vi "Write DAQmx Task Name.vi"(8 "error in (no error)":errorcluster, 10 "DAQmx Task Name":refnum<k21>, 11 "Pressure in":refnum<class "Pressure.lvclass">) -> (0 "error out":errorcluster, 3 "Pressure out":refnum<class "Pressure.lvclass">)   [LabVIEW 2018, in "Pressure Actor.lvlib" / "Pressure.lvclass"]
uses:
  Pressure.lvclass
  Pressure.lvclass/Pressure.ctl
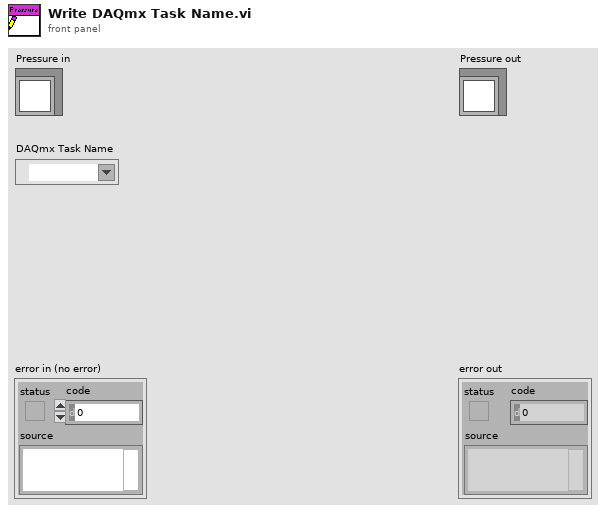
[diagram p1: front panel]
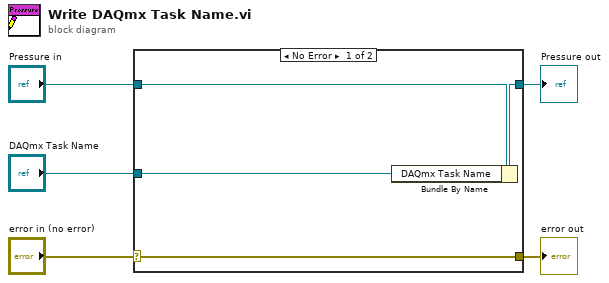
[diagram p0: block diagram]
diagram:
  n1 = case shown="No Error" "error in (no error)" {
    selector: "error in (no error)" -> [w9 w10]
    tunnel: [w9 w10] -> w4
    tunnel: [w7 w11] -> w2
    tunnel: "Pressure in" -> [w8 w11]
    tunnel: "DAQmx Task Name" -> [w6 _]
    frame No Error {
      n2 = Bundle By Name(cluster=w8, "DAQmx Task Name"=w6) -> (w7:refnum<class "Pressure.lvclass">)
    }
    frame Error {
    }
  }
  "error out" <- w4
  "Pressure out" <- w2
